vi "User_Defined_Test_CountsToTheta.vi"() -> (3 "Unit Test Framework Results":T1)   [LabVIEW 2016]
doc: "Use this template to create a user-defined test VI. Define your test requirements and wire the results to the <b>Result (Test)</b> control. Do not modify the <b>Unit Test Framework Results</b> indicator."
uses:
  <vilib>/utf/common/utf_test_result_troll.ctl
  <vilib>/utf/common/utf_test_result.ctl
  <vilib>/utf/common/utf_test_result_failure.ctl
  <vilib>/utf/common/utf_test_comparison_operators.ctl
  <vilib>/utf/common/utf_vi_tag.ctl
  <vilib>/Control Software Solutions Ltd/UTF Helper/Type Defs/Result Labels.ctl
  <vilib>/Control Software Solutions Ltd/UTF Helper/SubVIs/UTF Double Equals.vi
  MyPAM Controller/controllerLibrary.lvlib
  <vilib>/Control Software Solutions Ltd/UTF Helper/Unit Test Helper.lvlib
  <vilib>/utf/NI_UnitTestFramework.lvlib
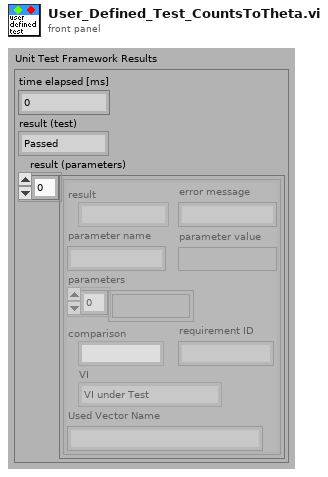
[diagram p1: front panel]
types:
  T1 = typedef "NI_UnitTestFramework.lvlib/utf_test_result_troll.ctl" = cluster{"time elapsed [ms]":u32, "result (test)":T2, "result (parameters)":T3[]}
  T2 = typedef "NI_UnitTestFramework.lvlib/utf_test_result.ctl" = enum16{"Passed", "Failed", "Error", "Skipped", "Not Processed"}
  T3 = typedef "NI_UnitTestFramework.lvlib/utf_test_result_failure.ctl" = cluster{"result":T2, "error message":string, "parameter name":string, "parameter value":variant, "parameters":variant[], "comparison":T4, "requirement ID":string, "VI":T5, "Used Vector Name":string}
  T4 = typedef "NI_UnitTestFramework.lvlib/utf_test_comparison_operators.ctl" = enum16{"=", "!=", ">", ">=", "<", "<=", "range", "symmetric tolerance", "asymmetric tolerance", "string contains", "string not contain", "array size", "string length", "array range", "by element", "array range (limit array)", "user-defined", "array contains", "array not contain", "vector length", "= (elm)", "!= (elm)", "= (case insensitive)", "!= (case insensitive)"}
  T5 = typedef "NI_UnitTestFramework.lvlib/utf_vi_tag.ctl" = enum16{"Setup VI", "VI under Test", "Teardown VI"}
  T6 = typedef "Unit Test Helper.lvlib/Result Labels.ctl" = cluster{"Requirement ID":string, "Error Message":string}
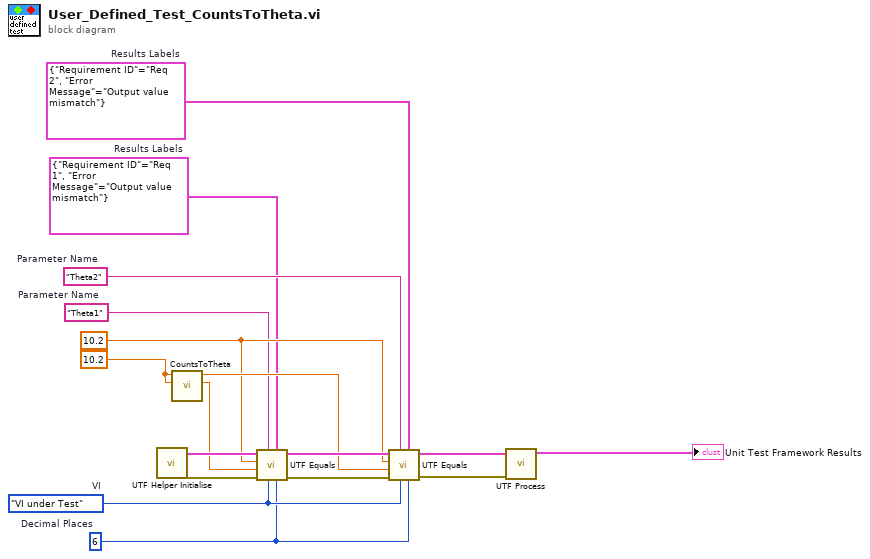
[diagram p0: block diagram]
diagram:
  w1 = T6 {"Requirement ID"="Req 2", "Error Message"="Output value mismatch"}  # Results Labels
  w2 = T6 {"Requirement ID"="Req 1", "Error Message"="Output value mismatch"}  # Results Labels
  w3 = u8 6  # Decimal Places
  w4 = utf_vi_tag."VI under Test"  # VI
  w5 = "Theta2"  # Parameter Name
  w6 = "Theta1"  # Parameter Name
  w7 = 10.2
  w10 = 10.2
  n1 = call <vilib>:"UTF Helper Initialise.vi"() -> ("error out"=w16:errorcluster, "results array"=w17:T3[])  [unwired: 10 in]
  n2 = call "CountsToTheta.vi"("Link2EncPos"=w10, "Link1EncPos"=w10) -> ("Theta1"=w9:dbl, "Theta0"=w8:dbl)  [unwired: 8 in]
  n3 = call-poly <vilib>:"UTF Equals.vi"("Decimal Places"=w3, "Results Labels"=w2, "VI"=w4, "Parameter Name"=w6, "error in (no error)"=w16, "Test Value"=w9, "Input"=w7, "Input Results"=w17) -> ("error out"=w14:errorcluster, "Output Results"=w15:T3[])  [unwired: 2 in]
  n4 = call-poly <vilib>:"UTF Equals.vi"("Decimal Places"=w3, "Results Labels"=w1, "VI"=w4, "Parameter Name"=w5, "error in (no error)"=w14, "Test Value"=w8, "Input"=w7, "Input Results"=w15) -> ("error out"=w12:errorcluster, "Output Results"=w13:T3[])  [unwired: 2 in]
  n5 = call <vilib>:"UTF Process.vi"("error in (no error)"=w12, "results array"=w13) -> ("Unit Test Framework Results"=→"Unit Test Framework Results":T1)  [unwired: 9 in]
